vi "Pack String to Long.vi"(4 "string":string) -> (1 "packed":u32[](array[numeric]) format="%.0b")   [LabVIEW 2011]
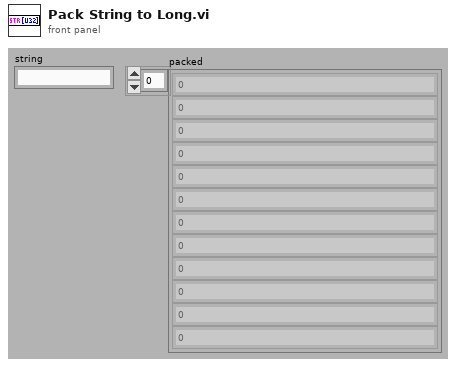
[diagram p1: front panel]
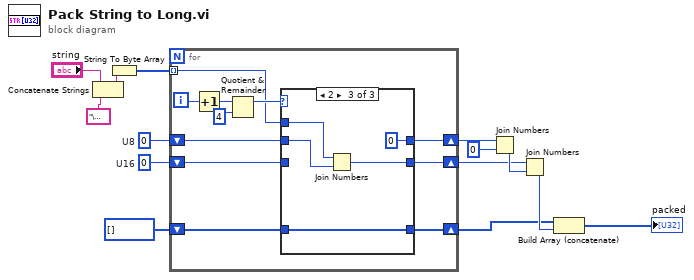
[diagram p0: block diagram]
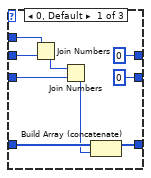
[diagram p2: hidden frame]
diagram:
  w10 = u16 0  # U16
  w11 = u8 0  # U8
  n1 = Concatenate Strings("string", "\u0000") -> (w13:string)
  n2 = String To Byte Array(string=w13) -> (unsigned byte array=w1:u8[])
  n3 = for {
    tunnel: w1 -> [w19] mode=indexing
    shift-right: [w25] -> w4
    shift-left: u32[] [] -> [w24]
    shift-right: [w18] -> w7
    shift-left: w11 -> [w17]
    shift-right: [w16] -> w6
    shift-left: w10 -> [w15]
    i -> [w23]
    n4 = Increment(x=w23) -> (x+1=w21:i32)
    n5 = Quotient & Remainder(x=w21, y=4) -> (x-y*floor(x/y)=w20:i32)  [unwired: 1 out]
    n6 = case shown="2" w20 {
      tunnel: [w31 w37 w42] -> w25
      tunnel: w24 -> [w32 w37 w42]
      tunnel: w19 -> [w28 w36 w38]
      tunnel: [u8 0 w36 u8 0] -> w18
      tunnel: w17 -> [w29 _ w39]
      tunnel: [u16 0 ("U16") w35 w40] -> w16
      tunnel: w15 -> [w27 w35 _]
      frame 0, Default {
        n7 = Join Numbers(hi=w28, lo=w29) -> ((hi.lo)=w26:u16)
        n8 = Join Numbers(hi=w26, lo=w27) -> ((hi.lo)=w30:u32)
        n9 = Build Array (concatenate)(w32, w30) -> (w31:u32[])
      }
      frame 1, 3 {
      }
      frame 2 {
        n10 = Join Numbers(hi=w38, lo=w39) -> ((hi.lo)=w40:u16)
      }
    }
  }
  n11 = Join Numbers(hi=w7, lo=u8 0) -> ((hi.lo)=w9:u16)
  n12 = Join Numbers(hi=w6, lo=w9) -> ((hi.lo)=w5:u32)
  n13 = Build Array (concatenate)(w4, w5) -> (→"packed":u32[])
